vi "Initialize.vi"(8 "error in":errorcluster, 10 "resource":string, 11 "host in":refnum<class "LIA Debugging Slow.lvclass">) -> (0 "error out":errorcluster, 3 "host out":refnum<class "LIA Debugging Slow.lvclass">)   [LabVIEW 2018, in "LIA Debugging Slow.lvclass"]
uses:
  LIA Debugging Slow.lvclass
  C:/Users/jfernand/Repositories/Lock-In-Amplifier/Shared/lib/interface/Interface FPGA/LIA Host Interface FPGA.lvclass
  Shared/lib/interface/Interface FPGA/Public/Session Data.ctl
  Shared/lib/interface/Interface FPGA/LIA Host Interface FPGA.lvclass/LIA Host Interface FPGA.ctl
  <vilib>/FPGAPlugInAG/PXIe-7976R/niLvFpga_Open_PXIe-7976R.vi
  <vilib>/rvi/interface/common/dynamic/niFpgaDynamicAddResources.vi
  <vilib>/Utility/error.llb/Error Cluster From Error Code.vi
  <vilib>/rvi/errors/niLvFpgaAdjustHostInterfaceError.vi
  <vilib>/rvi/interface/common/niFpgaWaitOnOcc.vi
  <vilib>/rvi/interface/nirviOpenFPGA/nirviOpenFPGA.xnode
  FPGA Bitfiles/LIA Debugging Slow FPGA.lvbitx
  <vilib>/rvi/interface/nirviReadWriteControl/nirviReadWriteControl.xnode
  <vilib>/rvi/interface/nirviMethod/nirviMethod.xnode
  Shared/lib/host/Lock-In Amplifier Example Host.lvlib
  Shared/lib/interface/Interface FPGA/LIA Host Interface FPGA.lvclass
  NiFpgaLv.dll
  <vilib>/rvi/interface/Simulation/niFpgaSimulationCallBeginRW.vi
  <vilib>/FPGAPlugInAG/Dynamic/niLvFpga_ConfigureFifo_Dynamic.vi
  <vilib>/rvi/errors/niLvFpgaMergeErrorWithErrorCode.vi
panel:
  out "Actual Depth":u32
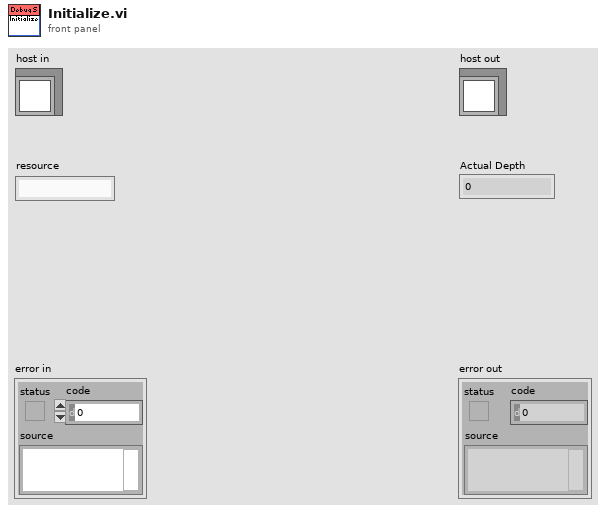
[diagram p1: front panel]
types:
  T1 = typedef "LIA Host Interface FPGA.lvclass/Session Data.ctl" = cluster{"fpga session":refnum<k20>, "record length":u32[]}
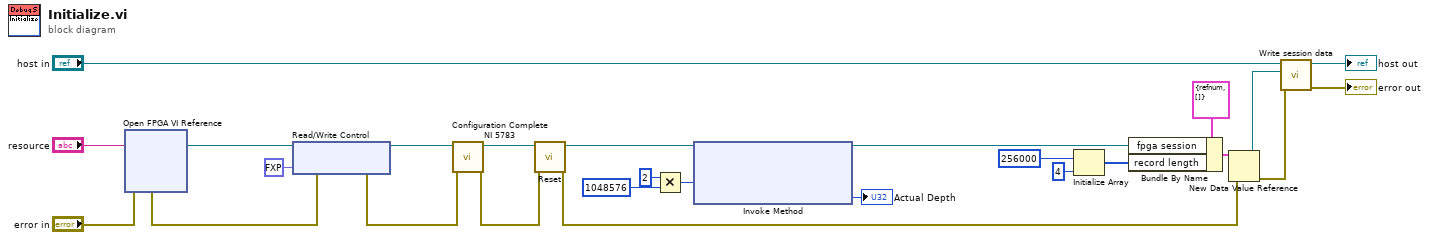
[diagram p0: block diagram]
diagram:
  n1 = xnode "Open FPGA VI Reference"("error in"="error in", "resource name"="resource") -> ("FPGA VI Reference Out"=w22:refnum<k20>, "error out"=w18:errorcluster)
  n2 = xnode "Read/Write Control"("FPGA VI Reference In"=w22, "error in"=w18, "ao.noise gain 3"=fxp<+,18,1> 0.0) -> ("FPGA VI Reference Out"=w19:refnum<k20>, "error out"=w17:errorcluster)
  n3 = call "Configuration Complete NI 5783.vi"("error in"=w17, "fpga session in"=w19) -> ("error out"=w21:errorcluster, "fpga session out"=w20:refnum<k20>)  [unwired: 7 in, 1 out]
  n4 = call "Reset.vi"("error in"=w21, "fpga session in"=w20) -> ("error out"=w23:errorcluster, "fpga session out"=w26:refnum<k20>)  [unwired: 8 in]
  n5 = Multiply(x=u32 2, y=u32 1048576 ("Requested Depth")) -> (x*y=w2:u32)
  n6 = xnode "Invoke Method"("FPGA VI Reference In"=w26, "Requested Depth"=w2) -> ("FPGA VI Reference Out"=w5:refnum<k20>, "Actual Depth"=→"Actual Depth":u32)  [unwired: 1 in, 1 out]
  n7 = Initialize Array(u32 256000 ("element"), 4 ("dimension size")) -> (w13:u32[])
  n8 = Bundle By Name(cluster=T1 {"fpga session"=refnum, "record length"=[]} ("session data"), "fpga session"=w5, "record length"=w13) -> (w24:T1)
  n9 = New Data Value Reference(data value=w24, error in=w23) -> (data value reference=w12:refnum<data-value>, error out=w11:errorcluster)
  n10 = call "Write session data.vi"("error in (no error)"=w11, "session data"=w12, "LIA Host Interface FPGA in"="host in") -> ("error out"=→"error out":errorcluster, "LIA Host Interface FPGA out"=→"host out":refnum<class "LIA Debugging Slow.lvclass">)  [unwired: 7 in]
